vi "SDI Init SDI.vi"(8 "error in (no error)":errorcluster, 9 "SDIIndex":u8, 10 "DevIndex":i32, 11 "DevType":i32) -> (0 "error out":errorcluster, 3 "function return":i32)   [LabVIEW 2012, in "ControlSDI.lvlib"]
doc: "int WINAPI SDI_InitSDI(int DevType, int DevIndex, unsigned char SDIIndex);"
uses:
  ControlSDI.lvlib
  Ginkgo_Driver.dll
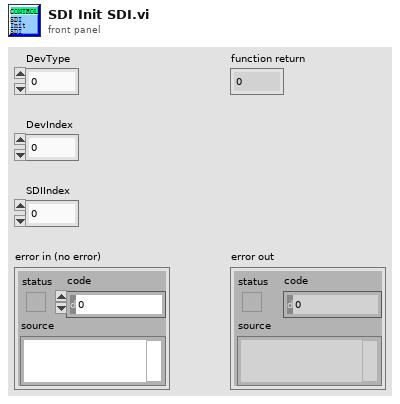
[diagram p1: front panel]
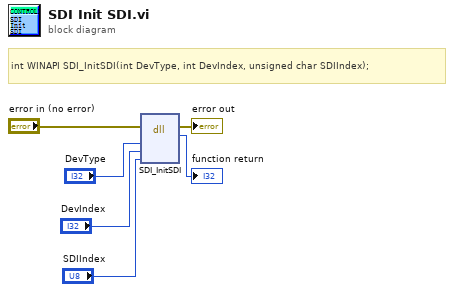
[diagram p0: block diagram]
diagram:
  # "int WINAPI SDI_InitSDI(int DevType, int DevIndex, unsigned char SDIIndex);"
  n1 = dll-call lib="E:/Project/vt_ginkgo/truck/Ginkgo Driver/vs2010/Ginkgo_USB-I2C_API_v2.0.3.0/lib/labview_32bit/ControlSDI/Ginkgo_Driver.*" fn="SDI_InitSDI"(error in="error in (no error)", "DevType"="DevType", "DevIndex"="DevIndex", "SDIIndex"="SDIIndex") -> (error out=→"error out":errorcluster, →"function return":i32)  [unwired: 5 in, 1 out]
